vi "Datatxt.vi"(0 "Объем скелета . см3":dbl format="%#.6f", 4 "Плотность зерен г/см3":dbl format="%#.6f", 5 "Наименование образца":string, 6 "Плотность образца.\n г/см3":dbl format="%#.6f", 7 "string":string="Пористость", 8 "Масса":dbl, 9 "длина":dbl, 10 "Диаметр":dbl, 11 "Пористость":dbl format="%#.6f") -> (3 "appended array":string[](array[string]))   [LabVIEW 2018]
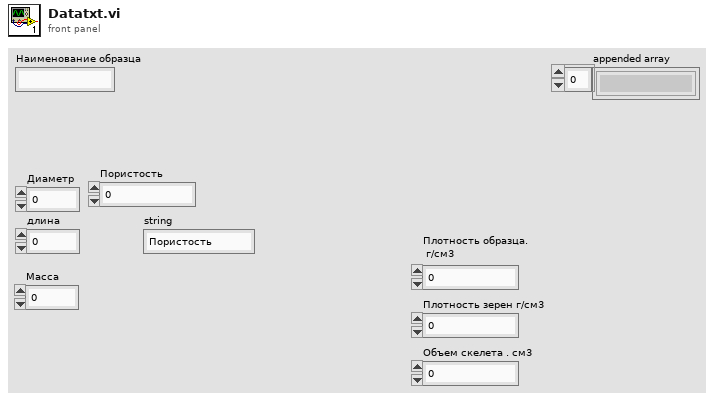
[diagram p1: front panel]
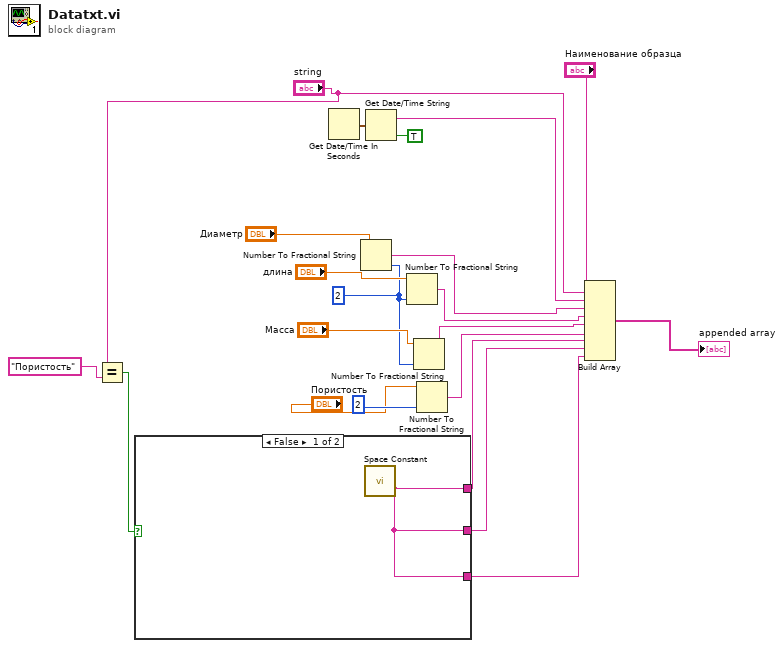
[diagram p0: block diagram]
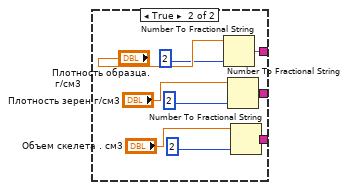
[diagram p2: hidden frame]
diagram:
  w12 = i16 2 ("precision (6)")
  n1 = Equal?(x="string", y="Пористость" ("string")) -> (x = y?=w2:bool)
  n2 = case shown="False" w2 {
    tunnel: [w22 w25] -> w7
    tunnel: [w22 w24] -> w6
    tunnel: [w22 w23] -> w5
    frame False {
      n3 = call <vilib>:"Space Constant.vi"() -> ("String"=w22:string)
    }
    frame True {
      n4 = Number To Fractional String(number="Плотность образца.\n г/см3", precision (6)=i16 2) -> (F-format string=w25:string)  [unwired: 2 in]
      n5 = Number To Fractional String(number="Плотность зерен г/см3", precision (6)=i16 2) -> (F-format string=w24:string)  [unwired: 2 in]
      n6 = Number To Fractional String(number="Объем скелета . см3", precision (6)=i16 2) -> (F-format string=w23:string)  [unwired: 2 in]
    }
  }
  n7 = Get Date/Time In Seconds() -> (seconds since 1Jan1904=w21:timestamp)
  n8 = Number To Fractional String(number="Диаметр", precision (6)=w12) -> (F-format string=w11:string)  [unwired: 2 in]
  n9 = Get Date/Time String(seconds (now)=w21, want seconds? (F)=TRUE) -> (date string=w15:string)  [unwired: 1 in, 1 out]
  n10 = Number To Fractional String(number="длина", precision (6)=w12) -> (F-format string=w10:string)  [unwired: 2 in]
  n11 = Number To Fractional String(number="Масса", precision (6)=w12) -> (F-format string=w9:string)  [unwired: 2 in]
  n12 = Number To Fractional String(number="Пористость", precision (6)=i16 2) -> (F-format string=w8:string)  [unwired: 2 in]
  n13 = Build Array("Наименование образца", "string", w15, w11, w10, w9, w8, w7, w6, w5) -> (→"appended array":string[])
